vi "Actor Core.vi"(8 "error in":errorcluster, 11 "DAQ970 in":refnum<class "DAQ970.lvclass">) -> (0 "error out":errorcluster, 3 "Actor out":refnum<class "Actor.lvclass">)   [LabVIEW 2019, in "DAQ970.lvlib" / "DAQ970.lvclass"]
doc: "The instrument actor core is only here to distribute panel resolution settings to children classes."
uses:
  Library/DAQ970.lvclass
  builds/Engine/Actor Framework.lvlibp/1abvi3w/vi.lib/ActorFramework/Actor/Actor.lvclass
  Custom Controls/Digital_In Control.ctl
  Custom Controls/Digital_Out Control.ctl
  Library/DAQ970.lvclass/DAQ970.ctl
  DAQ970 Messages/Toggle By Name Msg/Toggle By Name Msg.lvclass/Toggle By Name Msg.ctl
  Private/Accessors/Write Measured_Table_Ref.vi
  Private/Accessors/Write Display_Ref.vi
  builds/Engine/Actor Framework.lvlibp/1abvi3w/vi.lib/ActorFramework/Message Enqueuer/Enqueue.vi
  DAQ970 Messages/Toggle By Name Msg/Toggle By Name Msg.lvclass
  builds/Instruments/Instruments.lvlibp/Library/Instruments.lvclass
  builds/Instruments/Instruments.lvlibp/Instruments Messages/Measure Msg/Measure Msg.lvclass
  C:/Users/Public/Documents/Development/builds/Instruments/Instruments.lvlibp/Library/Instruments.lvclass
panel:
  in  "OK Button":bool
  in  "View":enum16{"Table", "Digital_Out", "Digital_In"}(ring)
  in  "Active Device":u16(ring)
  out "Tab Control":enum32{"Table", "Digital_Out", "Digital_In"}(tab)
  out "Measured Table":i32(listbox)
  in  "Digital_Out_3_Label":string[](array[string])
  in  "Digital_Out 3":T1
  in  "Digital_Out_2_Label":string[](array[string])
  in  "Digital_Out 2":T1
  in  "Digital_Out_1_Label":string[](array[string])
  in  "Digital_Out 1":T1
  in  "Digital_Out_0_Label":string[](array[string])
  in  "Digital_Out 0":T1
  out "Digital_In 3":T2
  in  "Digital_In_3_Label":string[](array[string])
  out "Digital_In 2":T2
  in  "Digital_In_2_Label":string[](array[string])
  out "Digital_In 1":T2
  in  "Digital_In_1_Label":string[](array[string])
  out "Digital_In 0":T2
  in  "Digital_In_0_Label":string[](array[string])
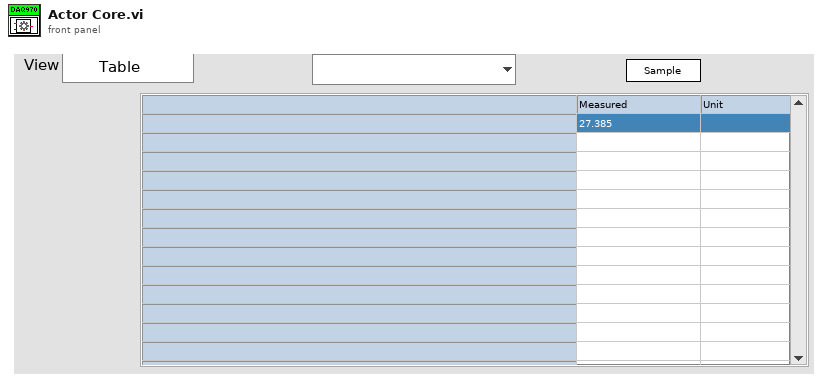
[diagram p1: front panel]
types:
  T1 = typedef "DAQ970.lvlib/DAQ970.lvclass/Digital_Out Control.ctl" = cluster{"DO 0":bool, "DO 1":bool, "DO 2":bool, "DO 3":bool, "DO 4":bool, "DO 5":bool, "DO 6":bool, "DO 7":bool}
  T2 = typedef "DAQ970.lvlib/DAQ970.lvclass/Digital_In Control.ctl" = cluster{"DI 0":bool, "DI 1":bool, "DI 2":bool, "DI 3":bool, "DI 4":bool, "DI 5":bool, "DI 6":bool, "DI 7":bool}
  T3 = cluster{"Pnl Actor":refnum<event-registration>, "Event Registration Refnum":refnum<event-registration>}
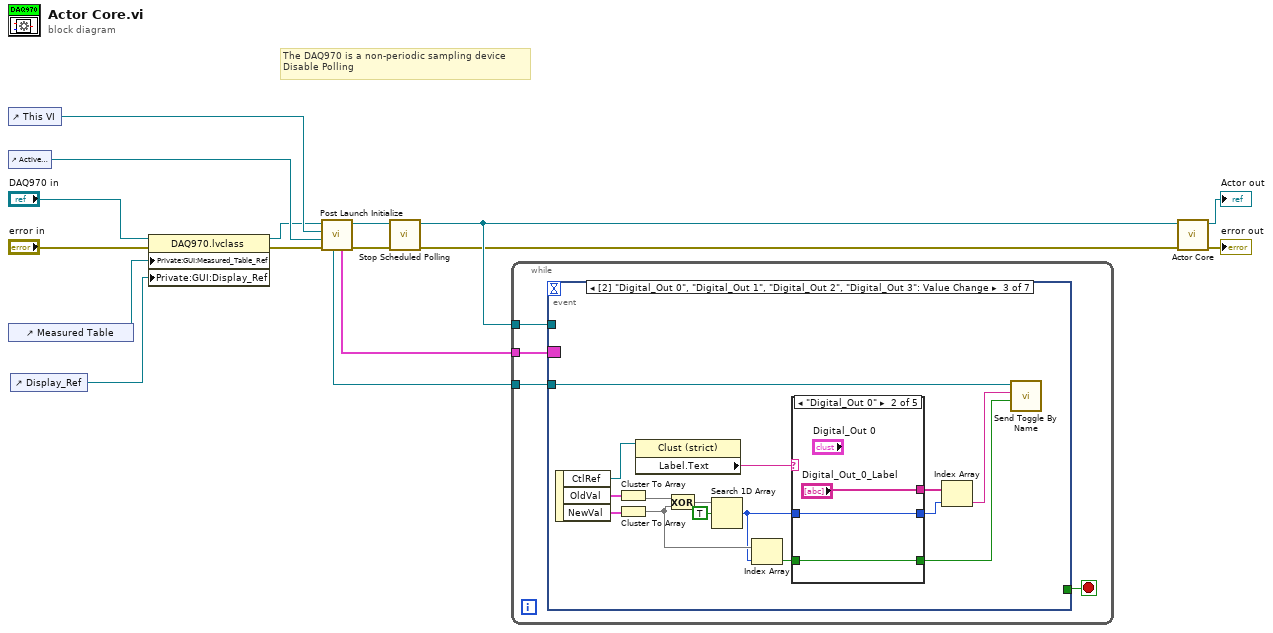
[diagram p0: block diagram]
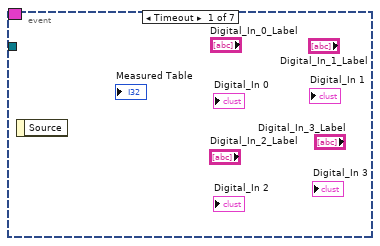
[diagram p2: hidden frame]
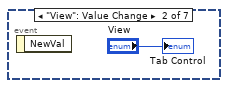
[diagram p3: hidden frame]
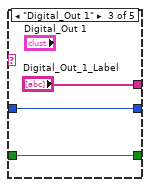
[diagram p5: hidden frame]
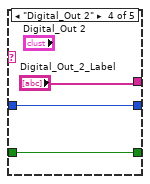
[diagram p6: hidden frame]
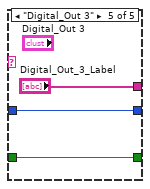
[diagram p7: hidden frame]
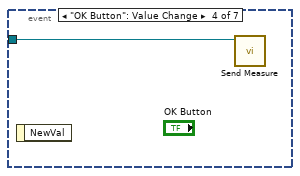
[diagram p8: hidden frame]
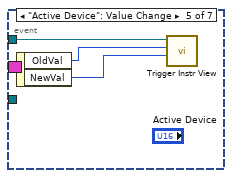
[diagram p9: hidden frame]
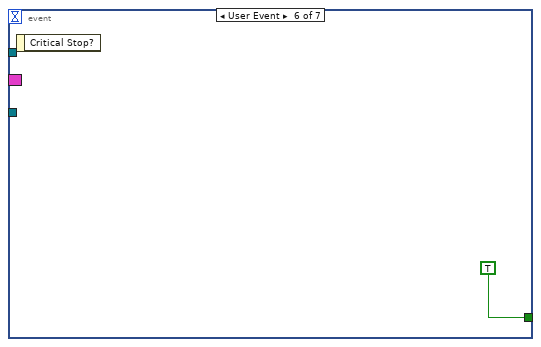
[diagram p10: hidden frame]
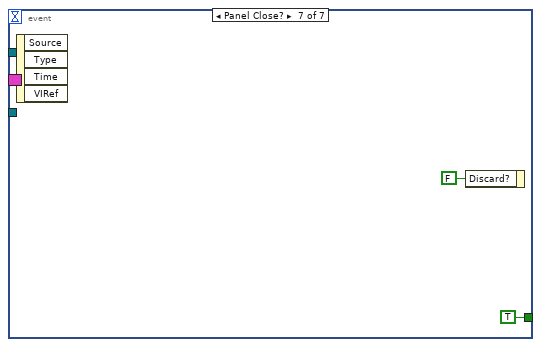
[diagram p11: hidden frame]
diagram:
  # "The DAQ970 is a non-periodic sampling device\nDisable Polling"
  n1 = control-ref of="This VI"() -> (w14:refnum<vi>)
  n2 = control-ref of="Active Device"() -> (w13:refnum<vi>)
  n3 = control-ref of="Measured Table"() -> (w6:refnum<vi>)
  n4 = control-ref of="Display_Ref"() -> (w1:refnum<vi>)
  n5 = property class="DAQ970.lvclass"(reference="DAQ970 in", error in="error in", "Private:GUI:Measured_Table_Ref"=w6, "Private:GUI:Display_Ref"=w1) -> (reference out=w9:refnum<class "DAQ970.lvclass">, error out=w7:errorcluster)
  n6 = call "Post Launch Initialize.vi"("error in"=w7, "Active Device"=w13, "GUI Reference"=w14, "Instruments in"=w9) -> ("error out"=w4:errorcluster, "Instruments out"=w5:refnum<class "DAQ970.lvclass">, "Registered Events"=w12:T3, "Self Enqueuer"=w11:refnum<class "Message Enqueuer.lvclass">)  [unwired: 4 in]
  n7 = call "Stop Scheduled Polling.vi"("error in"=w4, "Instruments in"=w5) -> ("error out"=w2:errorcluster, "Instruments out"=w3:refnum<class "DAQ970.lvclass">)  [unwired: 8 in]
  n8 = while {
    tunnel: w12 -> [w20]
    tunnel: w11 -> [w19]
    tunnel: w3 -> [w18]
    stop <- w17 stop-if-true
    n9 = event shown="[2] \"Digital_Out 0\", \"Digital_Out 1\", \"Digital_Out 2\", \"Digital_Out 3\": Value Change" {
      selector: w20 -> [_ _ _ _ _ _ _]
      dyn-events: _ -> [_ _ _ _ _ _ _]
      timeout: _ -> [_ _ _ _ _ _ _]
      tunnel: w19 -> [_ _ w24 w51 _ _ _]
      tunnel: w18 -> [_ _ _ _ w54 _ _]
      tunnel: [_ _ _ _ _ TRUE TRUE] -> w17
      event Timeout {
        n10 = event-data() -> ()  [unwired: 1 in, 1 out]
      }
      event "View": Value Change {
        n11 = event-data() -> ()  [unwired: 1 in, 1 out]
        "Tab Control" <- "View"
      }
      event Value Change {
        n12 = event-data() -> ("CtlRef"=w31:refnum<vi>, "OldVal"=w35:T1, "NewVal"=w36:T1)  [unwired: 1 in]
        n13 = Cluster To Array(cluster=w35) -> (array=w34:bool[])
        n14 = Cluster To Array(cluster=w36) -> (array=w29:bool[])
        n15 = property class="Clust (strict)"(reference=w31) -> ("Label.Text"=w30:string)  [unwired: 1 in, 2 out]
        n16 = Exclusive Or(1:w29, 2:w34) -> (0:w33:bool[])
        n17 = Search 1D Array(1D array=w33, element=TRUE) -> (index of element=w27:i32)  [unwired: 1 in]
        n18 = Index Array(array=w29, index=w27) -> (element=w28:bool)
        n19 = case shown="\"Digital_Out 0\"" w30 {
          tunnel: w28 -> [w37 w41 w44 w47 w50]
          tunnel: w27 -> [w38 w39 w43 w46 w49]
          tunnel: [w37 w41 w44 w47 w50] -> w22
          tunnel: [_ "Digital_Out_0_Label" "Digital_Out_1_Label" "Digital_Out_2_Label" "Digital_Out_3_Label"] -> w26
          tunnel: [w38 w39 w43 w46 w49] -> w25
          frame "False", Default {
          }
          frame "Digital_Out 0" {
          }
          frame "Digital_Out 1" {
          }
          frame "Digital_Out 2" {
          }
          frame "Digital_Out 3" {
          }
        }
        n20 = Index Array(array=w26, index=w25) -> (element=w23:string)
        n21 = call "Send Toggle By Name.vi"("State"=w22, "Name"=w23, "Message Enqueuer"=w24) -> ()  [unwired: 7 in, 2 out]
      }
      event "OK Button": Value Change {
        n22 = event-data() -> ()  [unwired: 1 in, 1 out]
        n23 = call "Send Measure.vi"("Message Enqueuer"=w51) -> ()  [unwired: 9 in, 2 out]
      }
      event "Active Device": Value Change {
        n24 = event-data() -> ("OldVal"=w53:u16, "NewVal"=w52:u16)  [unwired: 1 in]
        n25 = call "Trigger Instr View.vi"("New Value"=w52, "Old Value"=w53, "Instruments in"=w54) -> ()  [unwired: 7 in, 2 out]
      }
      event User Event {
        n26 = event-data() -> ()  [unwired: 1 in, 1 out]
      }
      event Panel Close? {
        n27 = event-data() -> ()  [unwired: 1 in, 4 out]
        n28 = event-data("Discard?"=FALSE) -> ()  [unwired: 1 in, 1 out]
      }
    }
  }
  n29 = call-parent "Actor Core.vi"("error in"=w2, "Instruments in"=w3) -> ("error out"=→"error out":errorcluster, "Actor out"=→"Actor out":refnum<class "Actor.lvclass">)  [unwired: 8 in]
